vi "Scale(Polynomial).vi"(10 "forward coeffs":dbl[](array[numeric]), 11 "unscaled value":dbl format="%#_13g") -> (3 "scale value":dbl)   [LabVIEW 2015, in "Scale.lvlib"]
uses:
  Scale.lvlib
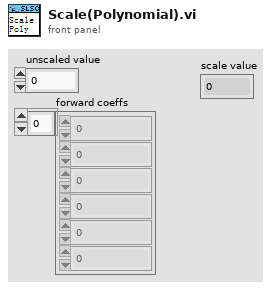
[diagram p1: front panel]
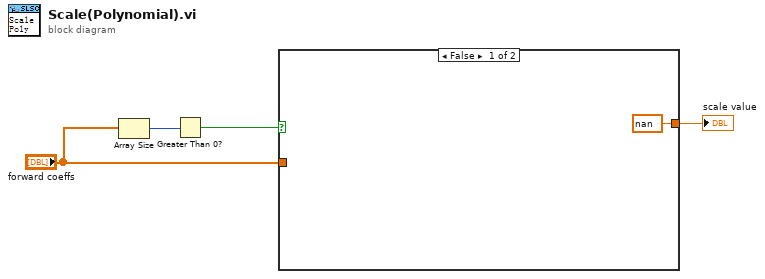
[diagram p0: block diagram]
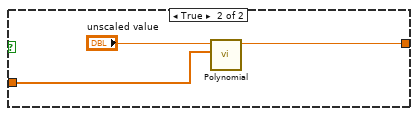
[diagram p2: hidden frame]
diagram:
  n1 = Array Size(array="forward coeffs") -> (size(s)=w4:i32)
  n2 = Greater Than 0?(x=w4) -> (x > 0?=w3:bool)
  n3 = case shown="False" w3 {
    tunnel: "forward coeffs" -> [_ w7]
    tunnel: [nan ("scaled value") w6] -> w1
    frame False {
    }
    frame True {
      n4 = call "Polynomial.vi"("coefficients"=w7, "init value"="unscaled value") -> ("scaled value"=w6:dbl)  [unwired: 9 in]
    }
  }
  "scale value" <- w1
